vi "10 Kwh battery decode.vi"(11 "String":string) -> (3 "Battery Data":string[](array[string]))   [LabVIEW 2021]
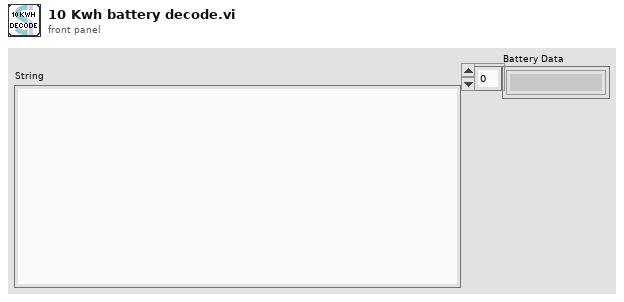
[diagram p1: front panel]
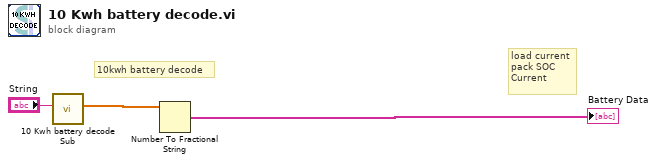
[diagram p0: block diagram]
diagram:
  # "load current\npack SOC\nCurrent"
  # "10kwh battery decode"
  n1 = call "10 Kwh battery decode Sub.vi"("Batter Data"="String") -> ("Data out"=w1:dbl[])  [unwired: 10 in]
  n2 = Number To Fractional String(number=w1) -> (F-format string=→"Battery Data":string[])  [unwired: 3 in]
